vi "GeraSinalEntreferro.vi"(0 "params":variant, 2 "Tx Aquisicao":dbl, 4 "estadoIn":variant) -> (15 "sinal":waveform(dbl), 18 "estadoOut":variant)   [LabVIEW 2017]
uses:
  Typedefs/Tipo_ParamsEntreferro.ctl
  Typedefs/Tipo_ComponenteSinalEntreferro.ctl
  <vilib>/Analysis/NI_AALBase.lvlib
panel:
  out "Waveform Graph":dbl[](graph)
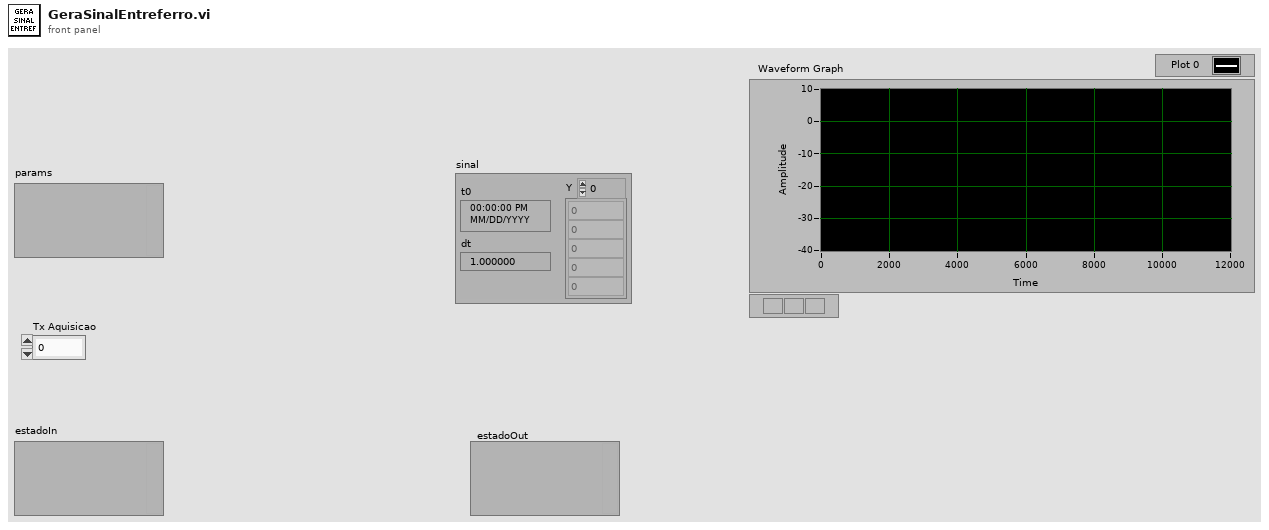
[diagram p1: front panel]
types:
  T1 = typedef "Tipo_ParamsEntreferro.ctl" = cluster{"Componentes":T2[], "Num Polos":u16, "Folga Nominal":dbl, "Ruido":dbl, "Saturacao":dbl, "Angulo":dbl}
  T2 = typedef "Tipo_ComponenteSinalEntreferro.ctl" = cluster{"Pólo:":u16, "Amplitude:":dbl}
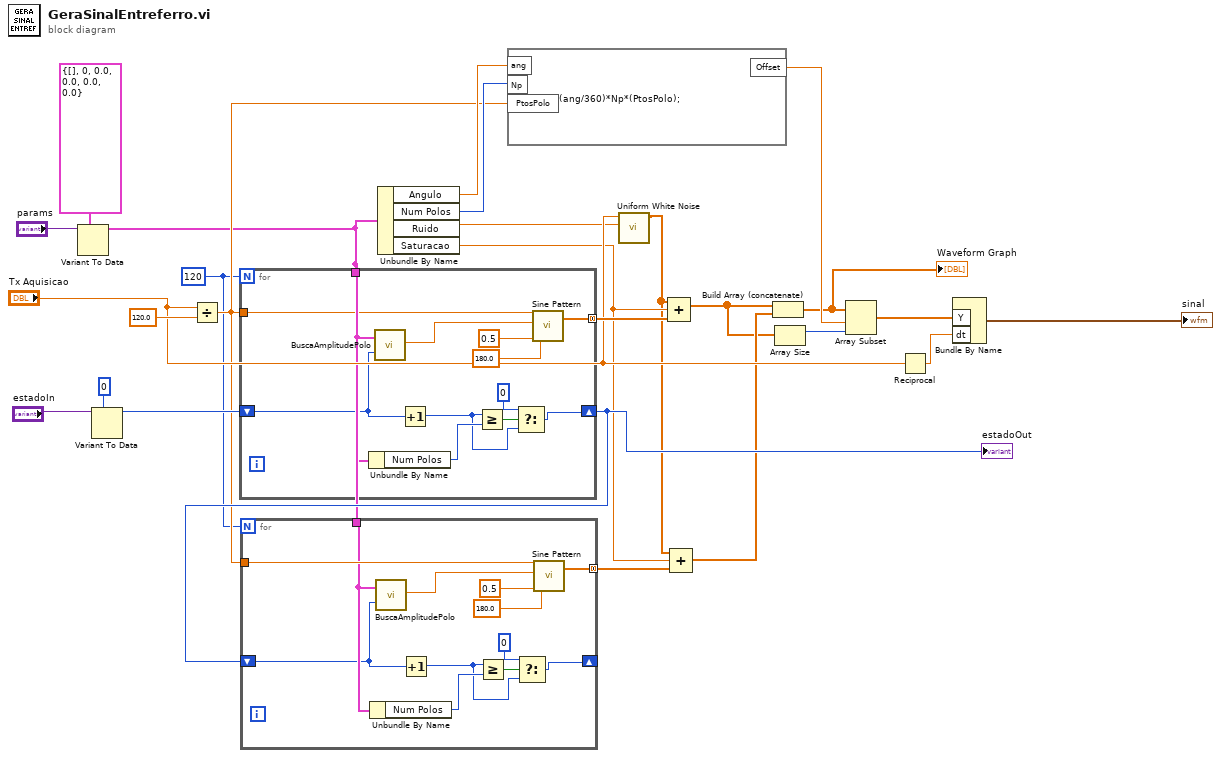
[diagram p0: block diagram]
diagram:
  w2 = 120
  n1 = Variant To Data(type=T1 {"Componentes"=[], "Num Polos"=0, "Folga Nominal"=0.0, "Ruido"=0.0, "Saturacao"=0.0, "Angulo"=0.0} ("Cluster"), Variant="params") -> (data=w11:T1)  [unwired: 1 in, 1 out]
  n2 = Variant To Data(type=u16 0, Variant="estadoIn") -> (data=w21:u16)  [unwired: 1 in, 1 out]
  n3 = Divide(x="Tx Aquisicao", y=120.0 ("x")) -> (x/y=w12:dbl)
  n4 = for {
    N: w2 -> [_]
    tunnel: w12 -> [w36]
    tunnel: [w35] -> w20 mode=concatenating
    tunnel: w11 -> [w33]
    shift-right: [w29] -> w13
    shift-left: w21 -> [w28]
    n5 = Unbundle By Name(w33) -> ("Num Polos"=w32:u16)
    n6 = call "BuscaAmplitudePolo.vi"("Config"=w33, "polo"=w28) -> ("Amp. Polo"=w34:dbl)  [unwired: 17 in]
    n7 = Increment(x=w28) -> (x+1=w27:u16)
    n8 = Greater Or Equal?(x=w27, y=w32) -> (x >= y?=w31:bool)
    n9 = Select(t=u16 0, s=w31, f=w27) -> (s? t:f=w29:u16)
    n10 = call <vilib>:"Sine Pattern.vi"("cycles"=0.5, "phase(degrees)"=180.0, "amplitude"=w34, "samples"=w36) -> ("Sinusoidal Pattern"=w35:dbl[])  [unwired: 1 out]
  }
  "estadoOut" <- w13
  n11 = for {
    N: w2 -> [_]
    tunnel: w12 -> [w48]
    tunnel: [w47] -> w10 mode=concatenating
    tunnel: w11 -> [w45]
    shift-right: [w41] -> _
    shift-left: w13 -> [w40]
    n12 = Unbundle By Name(w45) -> ("Num Polos"=w44:u16)
    n13 = call "BuscaAmplitudePolo.vi"("Config"=w45, "polo"=w40) -> ("Amp. Polo"=w46:dbl)  [unwired: 17 in]
    n14 = Increment(x=w40) -> (x+1=w39:u16)
    n15 = Greater Or Equal?(x=w39, y=w44) -> (x >= y?=w43:bool)
    n16 = Select(t=u16 0, s=w43, f=w39) -> (s? t:f=w41:u16)
    n17 = call <vilib>:"Sine Pattern.vi"("cycles"=0.5, "phase(degrees)"=180.0, "amplitude"=w46, "samples"=w48) -> ("Sinusoidal Pattern"=w47:dbl[])  [unwired: 1 out]
  }
  n18 = Unbundle By Name(w11) -> ("Angulo"=w14:dbl, "Num Polos"=w15:u16, "Ruido"=w16:dbl, "Saturacao"=w9:dbl)
  n19 = formula code="Offset = (ang/360)*Np*(PtosPolo);"("ang"=w14, "Np"=w15, "PtosPolo"=w12) -> ("Offset"=w6:dbl)
  n20 = call <vilib>:"Uniform White Noise.vi"("amplitude"=w16, "samples"="Tx Aquisicao") -> ("uniform white noise"=w8:dbl[])  [unwired: 8 in, 1 out]
  n21 = Compound Arithmetic op=ADD(w8, w9, w20) -> (w4:dbl[])
  n22 = Compound Arithmetic op=ADD(w8, w9, w10) -> (w7:dbl[])
  n23 = Build Array (concatenate)(w4, w7) -> (w1:dbl[])
  "Waveform Graph" <- w1
  n24 = Array Size(array=w4) -> (size(s)=w3:i32)
  n25 = Array Subset(array=w1, index=w6, length=w3) -> (w5:dbl[])
  n26 = Reciprocal(x="Tx Aquisicao") -> (1/x=w19:dbl)
  n27 = Bundle By Name("Y"=w5, "dt"=w19) -> (→"sinal":waveform(dbl))  [unwired: 1 in]
